vi "APC_9056_MergeCylErrors.vi"(5 "CylPressWarning":bool[][](array[boolean]), 9 "CylPressError":bool[][](array[boolean])) -> (4 "MaxPress":u8, 6 "Misfire (1 to 3)":u8, 8 "CyclicVar":u8, 10 "Knock":u8, 15 "LateComb":u8)   [LabVIEW 2020]
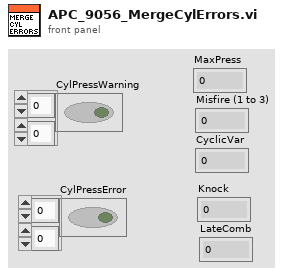
[diagram p1: front panel]
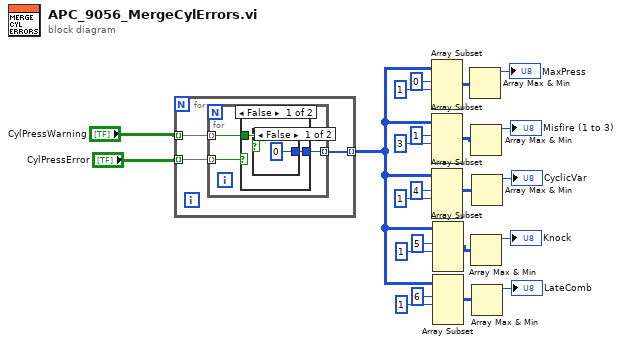
[diagram p0: block diagram]
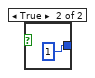
[diagram p2: hidden frame]
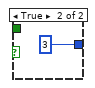
[diagram p3: hidden frame]
diagram:
  n1 = for {
    tunnel: "CylPressWarning" -> [w26] mode=indexing
    tunnel: "CylPressError" -> [w25] mode=indexing
    tunnel: [w24] -> w1 mode=indexing
    n2 = for {
      tunnel: w26 -> [w28] mode=indexing
      tunnel: w25 -> [w29] mode=indexing
      tunnel: [w27] -> w24 mode=indexing
      n3 = case shown="False" w29 {
        tunnel: [w30 3 ("length")] -> w27
        tunnel: w28 -> [w31 _]
        frame False {
          n4 = case shown="False" w31 {
            tunnel: [0 ("length") 1 ("length")] -> w30
            frame False {
            }
            frame True {
            }
          }
        }
        frame True {
        }
      }
    }
  }
  n5 = Array Subset(array=w1, index (row)=0 ("index"), length (row)=1 ("length")) -> (w13:i32[][])  [unwired: 2 in]
  n6 = Array Subset(array=w1, index (row)=1 ("index"), length (row)=3 ("length")) -> (w12:i32[][])  [unwired: 2 in]
  n7 = Array Subset(array=w1, index (row)=4 ("index"), length (row)=1 ("length")) -> (w11:i32[][])  [unwired: 2 in]
  n8 = Array Subset(array=w1, index (row)=5 ("index"), length (row)=1 ("length")) -> (w10:i32[][])  [unwired: 2 in]
  n9 = Array Subset(array=w1, index (row)=6 ("index"), length (row)=1 ("length")) -> (w9:i32[][])  [unwired: 2 in]
  n10 = Array Max & Min(array=w13) -> (max value=→"MaxPress":i32)  [unwired: 3 out]
  n11 = Array Max & Min(array=w12) -> (max value=→"Misfire (1 to 3)":i32)  [unwired: 3 out]
  n12 = Array Max & Min(array=w10) -> (max value=→"Knock":i32)  [unwired: 3 out]
  n13 = Array Max & Min(array=w11) -> (max value=→"CyclicVar":i32)  [unwired: 3 out]
  n14 = Array Max & Min(array=w9) -> (max value=→"LateComb":i32)  [unwired: 3 out]
